vi "Teleop.vi"(10 "Match Info":T1={"Autonomous Elapsed Seconds"=0.0, "TeleOp Elapsed Seconds"=0.0, "Disabled Elapsed Seconds"=0.0, "Visited Autonomous"=FALSE, "Visited TeleOp"=FALSE, "Visited Disabled"=FALSE, "Autonomous Settings"={"Autonomous Style"=enum."Independent", "VI Refnum"=refnum}}, 11 "Call Context":T2) -> ()   [LabVIEW 2017]
doc: "This VI is called for each TeleOp packet received from the DS where the robot is not disabled. It is often used to read from the joysticks and update I/O or to update setpoints for timed control loops. It should complete and return within 20 milliseconds or it may miss DS packets."
uses:
  <vilib>/Rock Robotics/WPI/DriverStation/WPI_DriverStationDerivedRobotMode.ctl
  <vilib>/Rock Robotics/WPI/DriverStation/WPI_DriverStationMatch Info.ctl
  <vilib>/Rock Robotics/WPI/ThirdParty/Phoenix-LabVIEW/Motor Controller/Controls/CTRE_Phoenix_MotorControl_ControlMode.ctl
  <vilib>/Rock Robotics/Network Tables/NT Read Boolean.vi
  <vilib>/Rock Robotics/Network Tables/NT Read Number.vi
  <vilib>/Rock Robotics/WPI/Utilities/WPI_GetSetVariantRefNum.vi
  <vilib>/Rock Robotics/WPI/ThirdParty/Phoenix-LabVIEW/Motor Controller/Get/CTRE_Phoenix_MotorController_GetSelectedSensorData.vi
panel:
  out "right":i32
  out "left":i32
  out "Sample Slider 0":dbl(slide) scale=0.0..5.0
  out "Sample Boolean 1":bool
  out "Sample Boolean 0":bool
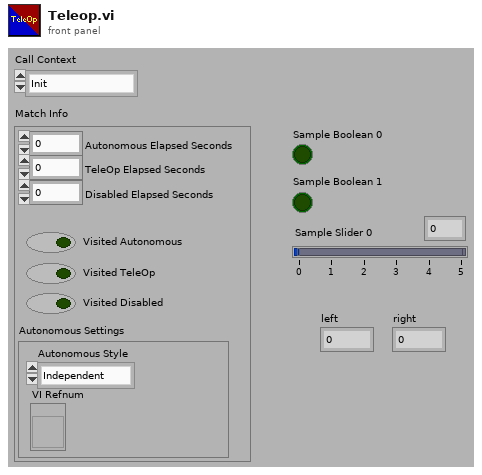
[diagram p1: front panel]
types:
  T1 = typedef "WPI_DriverStationMatch Info.ctl" = cluster{"Autonomous Elapsed Seconds":dbl, "TeleOp Elapsed Seconds":dbl, "Disabled Elapsed Seconds":dbl, "Visited Autonomous":bool, "Visited TeleOp":bool, "Visited Disabled":bool, "Autonomous Settings":cluster{"Autonomous Style":enum16{"Iterative", "Independent"}, "VI Refnum":refnum<vi>}}
  T2 = typedef "WPI_DriverStationDerivedRobotMode.ctl" = enum16{"Init", "Execute", "Stop"}
  T3 = typedef "CTRE_Phoenix_MotorControl_ControlMode.ctl" = u16
  T4 = typedef "WPI_MotorControlDeviceRef.ctl" = cluster{"DeviceStatus":errorcluster, "Type":T5, "PWM":cluster{"PWM Channel":T6, "DeadBand":T7}, "CAN":cluster{"Device Number":u8, "SetOutput VI Ref":variant, "GetOutput VI Ref":variant, "Enable VI Ref":variant, "Disable VI Ref":variant, "Data":variant}, "Invert":bool, "DIO PWM":cluster{"PWM \"Enable\" Channel":T6, "DIOChannel":T8, "PWM Rate":dbl}}
  T5 = typedef "WPI_MotorControlType.ctl" = enum16{"PWM", "CAN", "DIO PWM"}
  T6 = typedef "FPGA_DIOPWMChannel.ctl" = enum8{"PWM 0", "PWM 1", "PWM 2", "PWM 3", "PWM 4", "PWM 5", "PWM 6", "PWM 7", "PWM 8", "PWM 9", "PWM MXP 0", "PWM MXP 1", "PWM MXP 2", "PWM MXP 3", "PWM MXP 4", "PWM MXP 5", "PWM MXP 6", "PWM MXP 7", "PWM MXP 8", "PWM MXP 9", "Invalid"}
  T7 = typedef "WPI_PWMDeadband.ctl" = cluster{"Name":string, "maxPositivePwm":i32, "minPositivePwm":i32, "centerPwm":i32, "maxNegativePwm":i32, "minNegativePwm":i32, "angularRange":u16}
  T8 = typedef "FPGA_DIOChannel.ctl" = enum8{"DIO 0", "DIO 1", "DIO 2", "DIO 3", "DIO 4", "DIO 5", "DIO 6", "DIO 7", "DIO 8", "DIO 9", "DIO MXP 0", "DIO MXP 1", "DIO MXP 2", "DIO MXP 3", "DIO MXP 4", "DIO MXP 5", "DIO MXP 6", "DIO MXP 7", "DIO MXP 8", "DIO MXP 9", "DIO MXP 10", "DIO MXP 11", "DIO MXP 12", "DIO MXP 13", "DIO MXP 14", "DIO MXP 15", "SPI Port CS1", "SPI Port CS2", "SPI Port CS3", "SPI Port MISO", "SPI Port MOSI", "Invalid"}
  T9 = typedef "WPI_JoystickDevRef.ctl" = cluster{"Device":T10}
  T10 = typedef "WPI_JoystickDeviceEnum.ctl" = enum16{"USB 0", "USB 1", "USB 2", "USB 3", "USB 4", "USB 5"}
  T11 = typedef "WPI_SolenoidDevRef.ctl" = cluster{"DevStatus":errorcluster, "Pneumatics Control Module":u8, "Forward Solenoid Channel":T12, "Reverse Solenoid Channel":T12}
  T12 = typedef "WPI_SolenoidChannel.ctl" = enum8{"Solenoid 0", "Solenoid 1", "Solenoid 2", "Solenoid 3", "Solenoid 4", "Solenoid 5", "Solenoid 6", "Solenoid 7", "Invalid"}
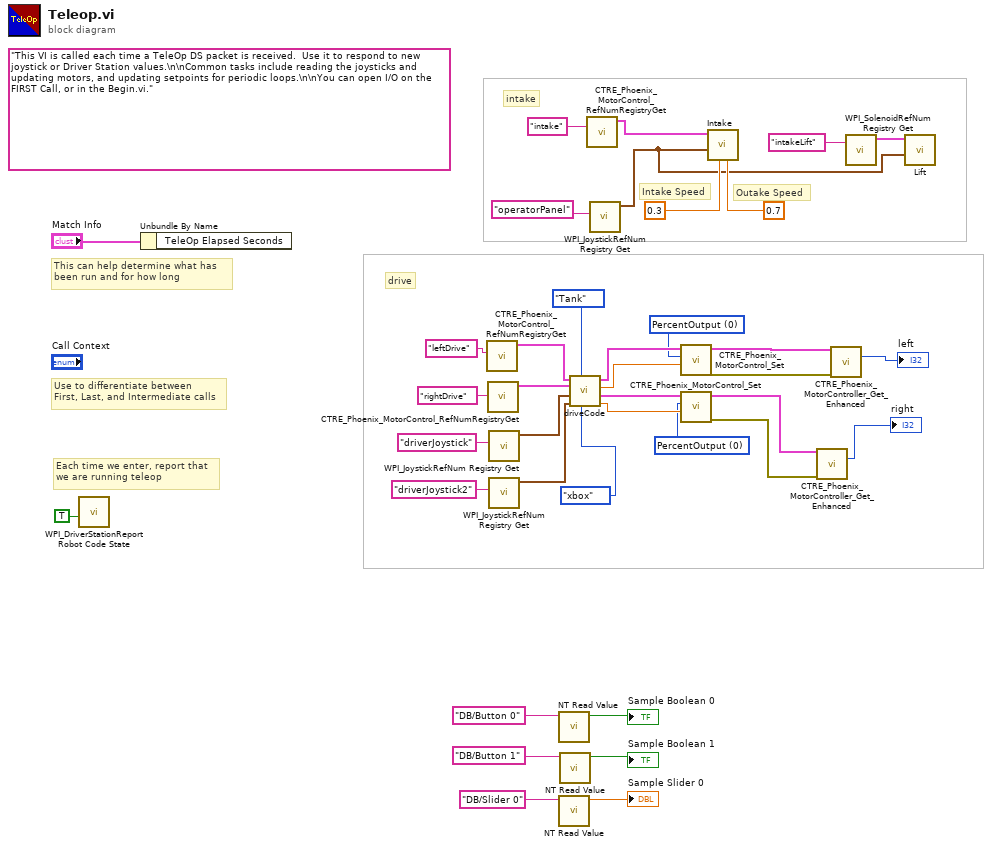
[diagram p0: block diagram]
diagram:
  w21 = T3 0 items=["PercentOutput"=0, "Position"=1, "Velocity"=2, "Current"=3, "Follower"=5, "MotionProfile"=6, "MotionMagic"=7, "MotionMagicArc"=8, "MotionProfileArc"=10, "Disabled"=15] ("Control Mode")
  w22 = T3 0 items=["PercentOutput"=0, "Position"=1, "Velocity"=2, "Current"=3, "Follower"=5, "MotionProfile"=6, "MotionMagic"=7, "MotionMagicArc"=8, "MotionProfileArc"=10, "Disabled"=15] ("Control Mode")
  (unwired) "This VI is called each time a TeleOp DS packet is received.  Use it to respond to new joystick or Driver Station values.\n\nCommon tasks include reading the joysticks and updating motors, and updating setpoints for periodic loops.\n\nYou can open I/O on the FIRST Call, or in the Begin.vi."
  # "drive"
  # "intake"
  # "Outake Speed"
  # "Intake Speed"
  # "Each time we enter, report that\nwe are running teleop"
  # "Use to differentiate between\nFirst, Last, and Intermediate calls"
  # "This can help determine what has\nbeen run and for how long"
  n1 = call <vilib>:"WPI_DriverStationReport Robot Code State.vi"("TeleOp"=TRUE ("Autonomous")) -> ()  [unwired: 10 in, 1 out]
  n2 = Unbundle By Name("Match Info") -> ()  [unwired: 1 out]
  n3 = call <vilib>:"CTRE_Phoenix_MotorControl_RefNumRegistryGet.vi"("refnum name"="leftDrive") -> ("PhoenixMotorControlDevRef"=w18:T4)  [unwired: 9 in, 1 out]
  n4 = call <vilib>:"CTRE_Phoenix_MotorControl_RefNumRegistryGet.vi"("refnum name"="rightDrive") -> ("PhoenixMotorControlDevRef"=w16:T4)  [unwired: 9 in, 1 out]
  n5 = call <vilib>:"WPI_JoystickRefNum Registry Get.vi"("refnum name"="driverJoystick") -> ("JoystickDevRef"=w30:T9)  [unwired: 9 in, 1 out]
  n6 = call <vilib>:"WPI_JoystickRefNum Registry Get.vi"("refnum name"="driverJoystick2") -> ("JoystickDevRef"=w29:T9)  [unwired: 9 in, 1 out]
  n7 = call-poly <vilib>:"NT Read Value.vi"("Name"="DB/Button 0" ("refnum name")) -> ("Boolean"=→"Sample Boolean 0":bool)  [unwired: 9 in, 1 out]
  n8 = call-poly <vilib>:"NT Read Value.vi"("Name"="DB/Slider 0" ("refnum name")) -> ("Numeric"=→"Sample Slider 0":dbl)  [unwired: 9 in, 1 out]
  n9 = call-poly <vilib>:"NT Read Value.vi"("Name"="DB/Button 1" ("refnum name")) -> ("Boolean"=→"Sample Boolean 1":bool)  [unwired: 9 in, 1 out]
  n10 = call "driveCode.vi"("tankJoystick"=enum16{"xbox", "twoJoystick"}."xbox", "mode"=enum16{"Tank", "Split Arcade", "Arcade"}."Tank", "driverJoystick2"=w29, "driverJoystick1"=w30, "rightDrive"=w16, "leftDrive"=w18) -> ("rightSpeed (%)"=w23:dbl, "rightDrive"=w25:T4, "leftSpeed (%)"=w24:dbl, "leftDrive"=w26:T4)  [unwired: 2 in]
  n11 = call <vilib>:"CTRE_Phoenix_MotorControl_RefNumRegistryGet.vi"("refnum name"="intake") -> ("PhoenixMotorControlDevRef"=w14:T4)  [unwired: 9 in, 1 out]
  n12 = call <vilib>:"WPI_JoystickRefNum Registry Get.vi"("refnum name"="operatorPanel") -> ("JoystickDevRef"=w1:T9)  [unwired: 9 in, 1 out]
  n13 = call <vilib>:"CTRE_Phoenix_MotorControl_Set.vi"("Output"=w24, "Control Mode"=w22, "PhoenixMotorControlDevRef"=w26) -> ("error out"=w8:errorcluster, "PhoenixMotorControlDevRef"=w9:T4)  [unwired: 7 in]
  n14 = call <vilib>:"CTRE_Phoenix_MotorControl_Set.vi"("Output"=w23, "Control Mode"=w21, "PhoenixMotorControlDevRef"=w25) -> ("error out"=w6:errorcluster, "PhoenixMotorControlDevRef"=w7:T4)  [unwired: 7 in]
  n15 = call "Intake.vi"("outakeSpeed"=0.7, "intakeSpeed"=0.3, "operatorPanel"=w1, "intake"=w14) -> ()  [unwired: 7 in, 1 out]
  n16 = call-poly <vilib>:"CTRE_Phoenix_MotorController_Get_Enhanced.vi"("PhoenixMotorControlDevRef"=w7, "error in"=w6) -> ("Position (Raw Sensor Units)"=→"right":i32)  [unwired: 10 in, 3 out]
  n17 = call-poly <vilib>:"CTRE_Phoenix_MotorController_Get_Enhanced.vi"("PhoenixMotorControlDevRef"=w9, "error in"=w8) -> ("Position (Raw Sensor Units)"=→"left":i32)  [unwired: 10 in, 3 out]
  n18 = call <vilib>:"WPI_SolenoidRefNum Registry Get.vi"("refnum name"="intakeLift") -> ("SolenoidDevRef"=w3:T11)  [unwired: 9 in, 1 out]
  n19 = call "Lift.vi"("operatorPanel"=w1, "intakeLift"=w3) -> ()  [unwired: 9 in, 1 out]
